vi "basic_encoder.vi"(8 "error in (no error)":errorcluster, 11 "Test Data in":T1) -> (0 "error out":errorcluster, 3 "Test Data out":T1)   [LabVIEW 2024, in "EncodingTester.lvlib"]
uses:
  EncodingTester.lvlib
  test_data--cluster.ctl
  packetized_data--cluster.ctl
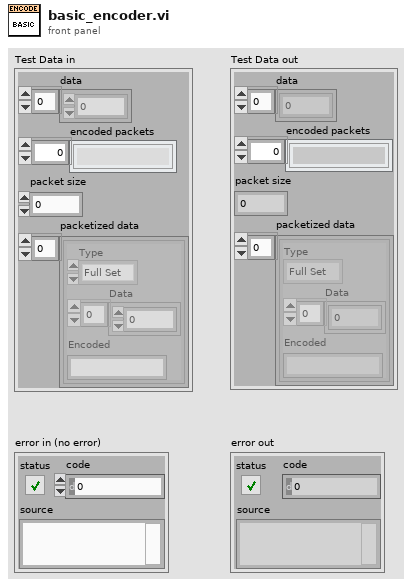
[diagram p1: front panel]
types:
  T1 = typedef "EncodingTester.lvlib/test_data--cluster.ctl" = cluster{"data":dbl[], "encoded packets":string[], "packet size":i32, "packetized data":T2[]}
  T2 = typedef "EncodingTester.lvlib/packetized_data--cluster.ctl" = cluster{"Type":enum16{"Full Set", "Last Set"}, "Data":dbl[], "Encoded":string}
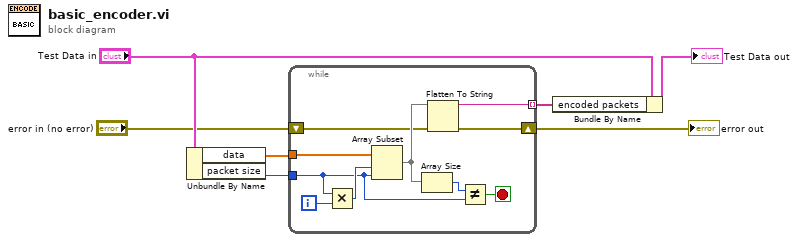
[diagram p0: block diagram]
diagram:
  n1 = Unbundle By Name("Test Data in") -> ("data"=w7:dbl[], "packet size"=w6:i32)
  n2 = while {
    tunnel: w7 -> [w17]
    tunnel: w6 -> [w13]
    tunnel: [w10] -> w5 mode=indexing
    shift-right: [w9] -> w1
    shift-left: "error in (no error)" -> [w8]
    i -> [w15]
    stop <- w11 stop-if-true
    n3 = Multiply(x=w13, y=w15) -> (x*y=w16:i32)
    n4 = Array Subset(array=w17, index=w16, length=w13) -> (w12:dbl[])
    n5 = Array Size(array=w12) -> (size(s)=w14:i32)
    n6 = Flatten To String(anything=w12, error in (no error)=w8) -> (data string=w10:string, error out=w9:errorcluster)  [unwired: 2 in, 1 out]
    n7 = Not Equal?(x=w14, y=w13) -> (x != y?=w11:bool)
  }
  "error out" <- w1
  n8 = Bundle By Name(cluster="Test Data in", "encoded packets"=w5) -> (→"Test Data out":T1)
